vi "get_all_collections.vi"(0 "vector_weviate in":refnum<class "vector_weviate.lvclass">, 11 "error in (no error)":errorcluster) -> (4 "vector_weviate out":refnum<class "vector_weviate.lvclass">, 6 "collection":string[](array[string]), 15 "error out":errorcluster)   [LabVIEW 2020, in "vector_weviate.lvclass"]
doc: "Gets all the collections from the Weviate vector store"
uses:
  vector_weviate.lvclass
  vector_weviate.lvclass/vector_weviate.ctl
  <vilib>/httpClient/LabVIEWHTTPClient.lvlib
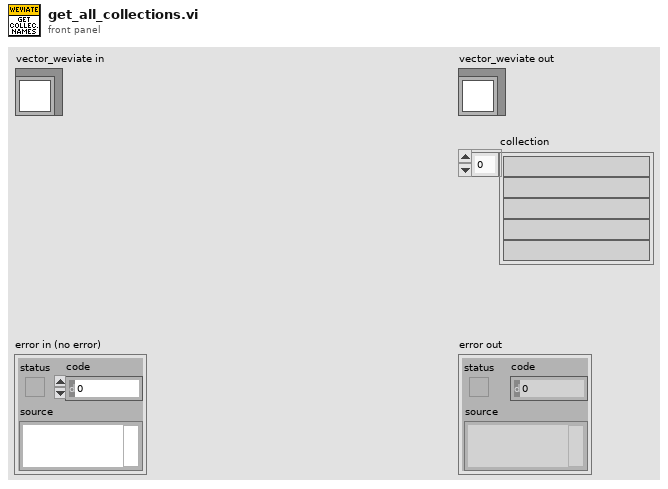
[diagram p1: front panel]
types:
  T1 = typedef "LabVIEWHTTPClient.lvlib/ClientHandle.ctl" = refnum<k1>
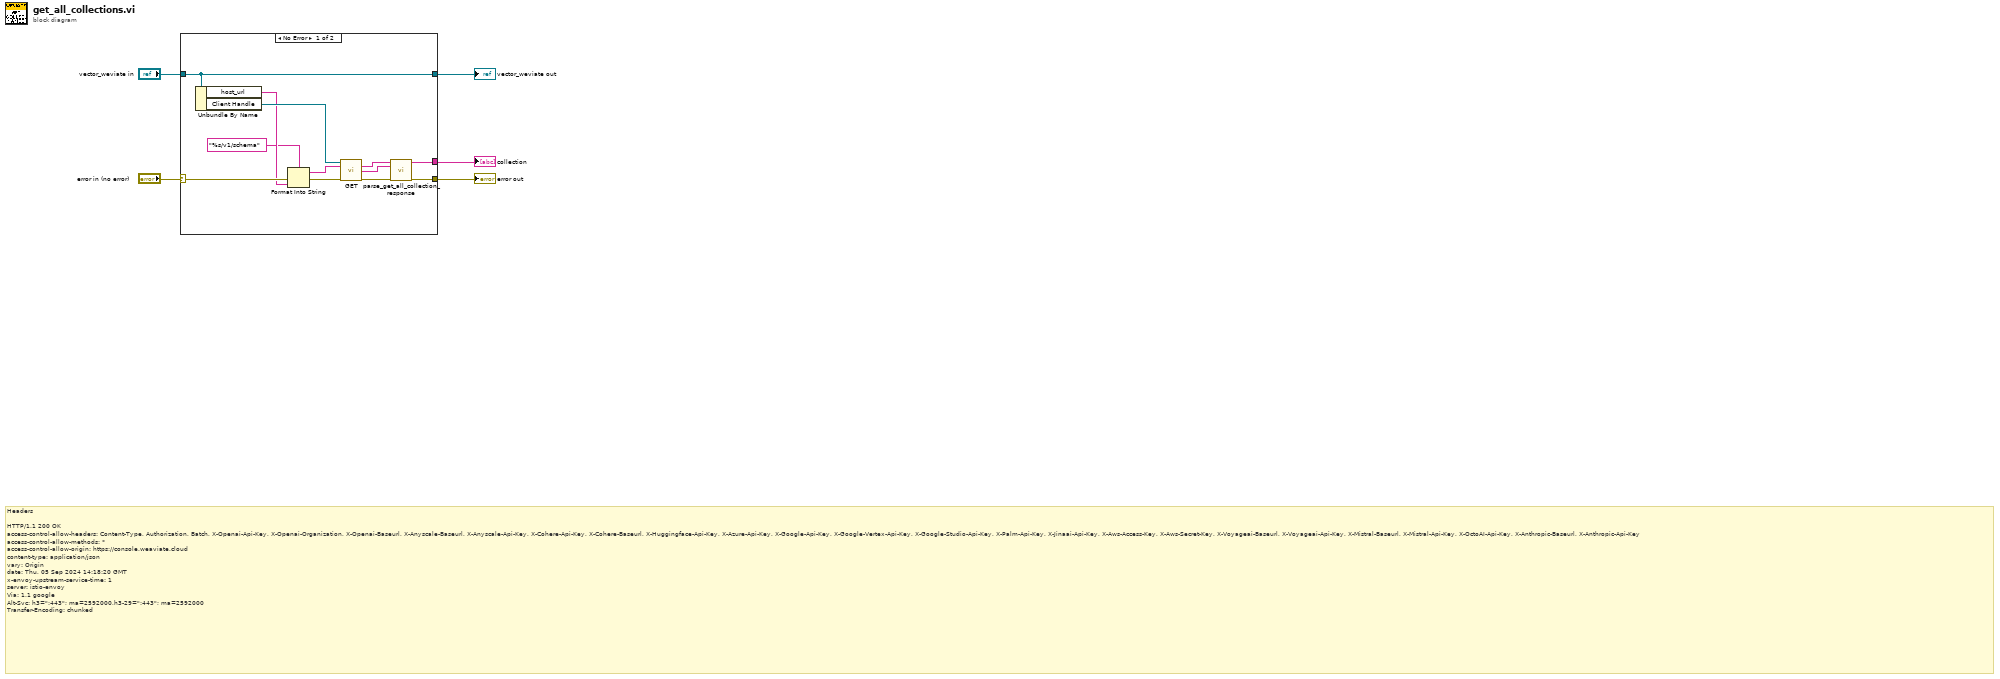
[diagram p0: block diagram]
diagram:
  # "Headers\n\nHTTP/1.1 200 OK\naccess-control-allow-headers: Content-Type, Authorization, Batch, X-Openai-Api-Key, X-Openai-Organization, X-Openai-Baseurl, X-Anyscale-Baseurl, X-Anyscale-Api-Key, X-Cohere-Api-Key, X-Cohere-Baseurl, X-Huggingface-Api-Key, X-Azure-Api-Key, X-Google-Api-Key, X-Google-Vertex-Api-Key, X-Google-Studio-Api-Key, X-Palm-Api-Key, X-Jinaai-Api-Key, X-Aws-Access-Key, X-Aws-Secret-Key, X-Voyageai-Baseurl, X-Voyageai-Api-Key, X-Mistral-Baseurl, X-Mistral-Api-Key, X-OctoAI-Api-Key, X-Anthropic-Baseurl, X-Anthropic-Api-Key\naccess-control-allow-methods: *\naccess-control-allow-origin: https://console.weaviate.cloud\ncontent-type: application/json\nvary: Origin\ndate: Thu, 05 Sep 2024 14:18:20 GMT\nx-envoy-upstream-service-time: 1\nserver: istio-envoy\nVia: 1.1 google\nAlt-Svc: h3=\":443\"; ma=2592000,h3-29=\":443\"; ma=2592000\nTransfer-Encoding: chunked"
  n1 = case shown="No Error" "error in (no error)" {
    selector: "error in (no error)" -> [w16 w18]
    tunnel: "vector_weviate in" -> [w11 w19]
    tunnel: [w11 w19] -> w3
    tunnel: [w7 w18] -> w2
    tunnel: [w6 _] -> w1
    frame No Error {
      n2 = Unbundle By Name(w11) -> ("host_url"=w14:string, "Client Handle"=w17:T1)
      n3 = Format Into String(format string="%s/v1/schema", error in=w16, w14) -> (resulting string=w12:string, error out=w15:errorcluster)  [unwired: 1 in]
      n4 = call <vilib>:"GET.vi"("client handle"=w17, "url"=w12, "error in (no error)"=w15) -> ("headers"=w9:string, "body"=w8:string, "error out"=w10:errorcluster)  [unwired: 9 in, 1 out]
      n5 = call "parse_get_all_collection_response.vi"("headers"=w9, "body"=w8, "error in (no error)"=w10) -> ("collection_list"=w6:string[], "error out"=w7:errorcluster)  [unwired: 11 in]
    }
    frame Error {
    }
  }
  "error out" <- w2
  "vector_weviate out" <- w3
  "collection" <- w1
